vi "自动垫片有无运行.vi"(0 "Image In":T1(plugin-control), 5 "error in (no error)":errorcluster caption="错误输入（无错误）") -> (14 "Image out":T1(plugin-control), 15 "铜片有/无":bool, 16 "异常":bool, 19 "error out":errorcluster caption="错误输出")   [LabVIEW 2017]
uses:
  Global System.vi
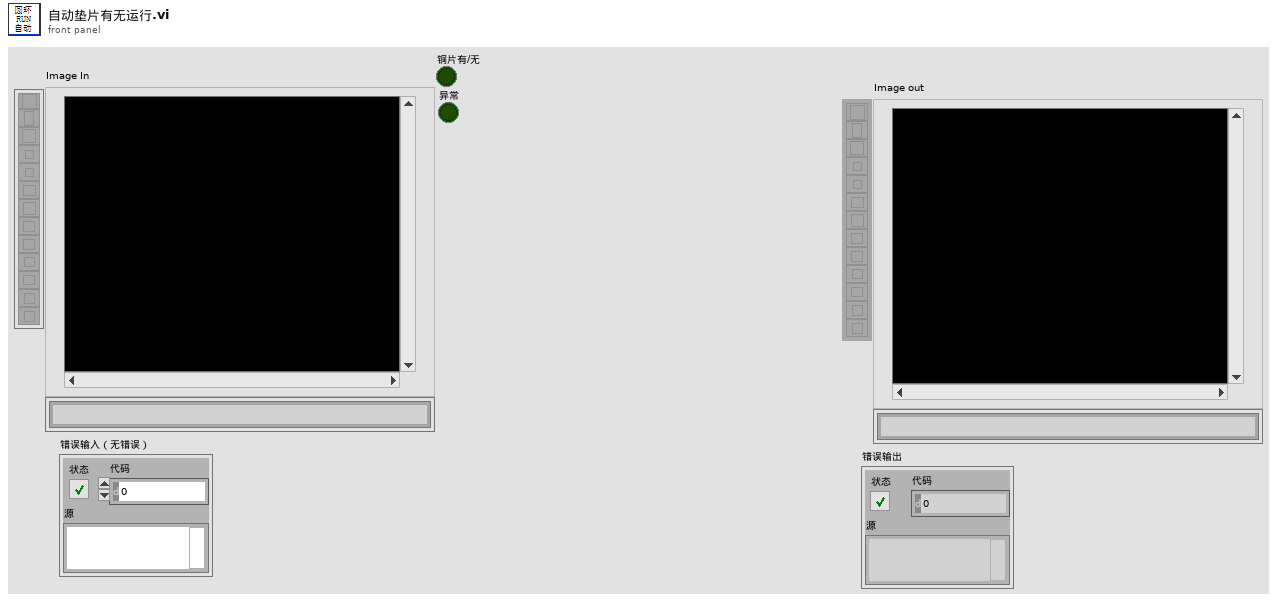
[diagram p1: front panel]
types:
  T1 = typedef "IMAQ Image.ctl" = refnum<image>
  T2 = typedef "IMAQ Circle" = cluster{"Center X":i32, "Center Y":i32, "Inner Radius":i32, "Outer Radius":i32, "Start Angle":dbl, "End Angle":dbl}
  T3 = typedef "ROI Descriptor" = cluster{"Global Rectangle":i32[], "Contours":cluster{"ID":enum32{"External", "Internal"}, "Type":u32, "Coordinates":i32[]}[]}
  T4 = cluster{"Center (Pixels)":cluster{"X":sgl, "Y":sgl}, "Radius (Pixels)":dbl, "Center (Real-World)":cluster{"X":sgl, "Y":sgl}, "Radius (Real-World)":dbl, "Roundness (Real-World)":dbl, "Average Strength":dbl, "Average SNR (dB)":dbl}
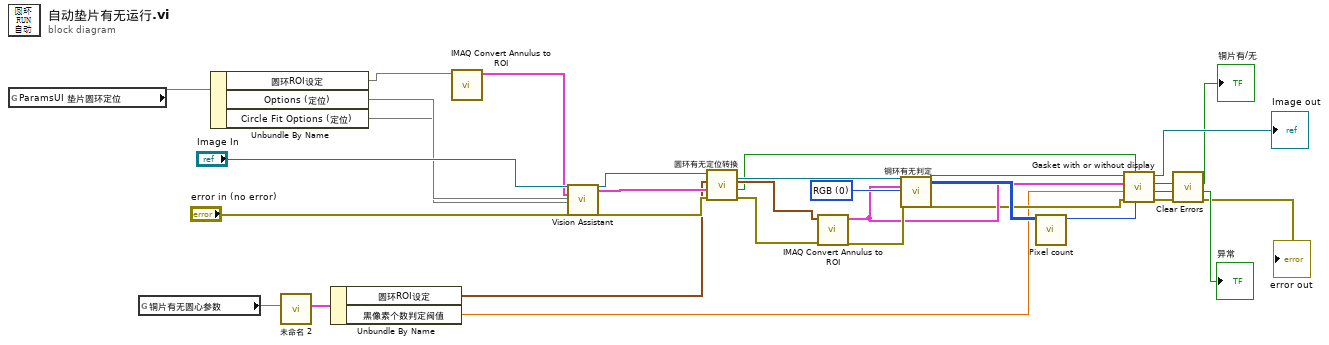
[diagram p0: block diagram]
diagram:
  w15 = u16 0 items=["RGB", "HSL", "HSV", "HSI"] ("Color Mode (Histogram 1)")
  n1 = global read "Global System.vi" "ParamsUI 垫片圆环定位"() -> (w28)
  n2 = global read "Global System.vi" "铜片有无圆心参数"() -> (w23)
  n3 = Unbundle By Name(w28) -> ("圆环ROI设定"=w27, "Options (定位)"=w25, "Circle Fit Options (定位)"=w24)
  n4 = call "未命名 2.vi"("铜片有无圆心参数"=w23) -> ("输出簇 2"=w22:cluster{"圆环ROI设定":T2, "黑像素个数判定阀值":dbl})  [unwired: 10 in]
  n5 = Unbundle By Name(w22) -> ("圆环ROI设定"=w18:T2, "黑像素个数判定阀值"=w8:dbl)
  n6 = call "IMAQ Convert Annulus to ROI"("Annulus"=w27) -> ("ROI Descriptor"=w26:T3)  [unwired: 8 in, 1 out]
  n7 = call "Vision Assistant"("Image In"="Image In", "ROI Descriptor (Find Circular Edge 1)"=w26, "Options (Find Circular Edge 1)"=w25, "Circle Fit Options (Find Circular Edge 1)"=w24, "error in"="error in (no error)") -> ("Image Out"=w19:T1, "Fitted Circle (Find Circular Edge 1)"=w21:T4, "error out"=w20:errorcluster)  [unwired: 20 in]
  n8 = call "圆环有无定位转换.vi"("error in (no error)"=w20, "Fitted Circle (定位)"=w21, "圆环ROI设定 in"=w18, "Image in"=w19) -> ("error out"=w10:errorcluster, "有无定位"=w2:bool, "圆环ROI设定 out"=w4:T2, "Image out"=w9:T1)  [unwired: 4 in]
  n9 = call "IMAQ Convert Annulus to ROI"("error in (no error)"=w10, "Annulus"=w4) -> ("error out"=w16:errorcluster, "ROI Descriptor"=w13:T3)  [unwired: 7 in]
  n10 = call "铜环有无判定"("Image In"=w9, "ROI Descriptor (Histogram 1)"=w13, "Color Mode (Histogram 1)"=w15, "error in"=w16) -> ("Image Out"=w17:T1, "Histogram (Histogram 1)"=w14:u32[][], "error out"=w12:errorcluster)  [unwired: 20 in, 1 out]
  n11 = call "Pixel count.vi"("Histogram 图标"=w14) -> ("像素黑个数"=w11:u32)  [unwired: 9 in, 1 out]
  n12 = call "Gasket with or without display.vi"("黑像个数"=w11, "有无定位"=w2, "error in (no error)"=w12, "黑像素阀值判定个数"=w8, "ROI Descriptor"=w13, "原始图像 IN"=w17) -> ("error out"=w6:errorcluster, "异常"=→"异常":bool, "铜片有/无"=→"铜片有/无":bool, "原始图像 OUT"=→"Image out":T1)  [unwired: 2 in]
  n13 = call <vilib>:"Clear Errors.vi"("error in (no error)"=w6) -> ("error out"=→"error out":errorcluster)  [unwired: 5 in, 1 out]
